vi "Drive Controller.vi"(8 "error in":errorcluster) -> ()   [LabVIEW 2018]
doc: "This VI executes continuously carrying out the current operation and responding to updates or new operation requests. It will often contain the timing or control code that is difficult to place directly in TeleOp. This VI generally opens all sensors and motors and isolates the rest of the robot code from knowing implementation details of how the operations are carried out."
uses:
  <vilib>/Rock Robotics/WPI/Framework/Completion Status.ctl
  Drive Setpoints.ctl
  Drive Operations.ctl
  <vilib>/Rock Robotics/WPI/SafetyOutput/WPI_SafetyOutputConfigMenu.ctl
  <vilib>/Rock Robotics/WPI/RobotDrive/WPI_RobotDriveOpen2MotorWithExistingMotors.vi
  <vilib>/Rock Robotics/Network Tables/NT Write Number.vi
panel:
  in  "Interactive Values":T1
  in  "Buttons":cluster{"Execute Cmd":bool, "Abort Cmd":bool}
  out "Command Timing":cluster{"Start Time (ms)":u32, "Iterations":i32}
  out "Status":T3
  out "Setpoints":T4(graph)
  out "Current\nCmd":string
  # "Tip: The graph shows the motor setpoints. It may also be helpful to observe inputs and sensor values.\nYou may also want to display tuning or debugging controls."
  # "Interactive Command: You may fill in the settings for a command\nand schedule it with the Execute button. You can observe and abort\nany command while fine tuning the code for the controller."
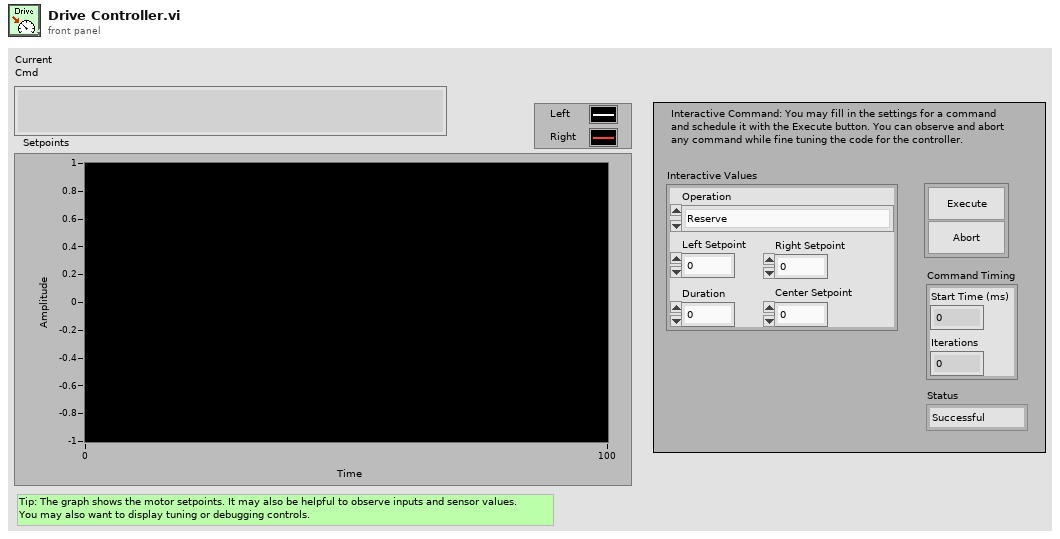
[diagram p1: front panel]
types:
  T1 = typedef "Drive Setpoints.ctl" = cluster{"Operation":T2, "Left Setpoint":dbl, "Right Setpoint":dbl, "Duration":dbl, "Center Setpoint":dbl}
  T2 = typedef "Drive Operations.ctl" = enum16{"Reserve", "Read Current", "Immediate", "Drive for Time", "Drive for Distance"}
  T3 = typedef "Completion Status.ctl" = enum16{"Successful", "Aborted", "Incomplete"}
  T4 = cluster{"Don't move motors while reserved":dbl, "Don't move motors while reserved":dbl, "Center Setpoint":dbl}
  T5 = typedef "WPI_SafetyOutputConfigMenu.ctl" = enum16{"Enable", "Disable"}
  T6 = typedef "WPI_MotorControlDeviceRef.ctl" = cluster{"DeviceStatus":errorcluster, "Type":T7, "PWM":cluster{"PWM Channel":T8, "DeadBand":T9}, "CAN":cluster{"Device Number":u8, "SetOutput VI Ref":variant, "GetOutput VI Ref":variant, "Enable VI Ref":variant, "Disable VI Ref":variant, "Data":variant}, "Invert":bool, "DIO PWM":cluster{"PWM \"Enable\" Channel":T8, "DIOChannel":T10, "PWM Rate":dbl}}
  T7 = typedef "WPI_MotorControlType.ctl" = enum16{"PWM", "CAN", "DIO PWM"}
  T8 = typedef "FPGA_DIOPWMChannel.ctl" = enum8{"PWM 0", "PWM 1", "PWM 2", "PWM 3", "PWM 4", "PWM 5", "PWM 6", "PWM 7", "PWM 8", "PWM 9", "PWM MXP 0", "PWM MXP 1", "PWM MXP 2", "PWM MXP 3", "PWM MXP 4", "PWM MXP 5", "PWM MXP 6", "PWM MXP 7", "PWM MXP 8", "PWM MXP 9", "Invalid"}
  T9 = typedef "WPI_PWMDeadband.ctl" = cluster{"Name":string, "maxPositivePwm":i32, "minPositivePwm":i32, "centerPwm":i32, "maxNegativePwm":i32, "minNegativePwm":i32, "angularRange":u16}
  T10 = typedef "FPGA_DIOChannel.ctl" = enum8{"DIO 0", "DIO 1", "DIO 2", "DIO 3", "DIO 4", "DIO 5", "DIO 6", "DIO 7", "DIO 8", "DIO 9", "DIO MXP 0", "DIO MXP 1", "DIO MXP 2", "DIO MXP 3", "DIO MXP 4", "DIO MXP 5", "DIO MXP 6", "DIO MXP 7", "DIO MXP 8", "DIO MXP 9", "DIO MXP 10", "DIO MXP 11", "DIO MXP 12", "DIO MXP 13", "DIO MXP 14", "DIO MXP 15", "SPI Port CS1", "SPI Port CS2", "SPI Port CS3", "SPI Port MISO", "SPI Port MOSI", "Invalid"}
  T11 = typedef "WPI_RobotDriveDevRef.ctl" = cluster{"DevStatus":errorcluster, "Motors[]":T6[], "Square Inputs":bool, "Max Output":dbl}
  T12 = typedef "Command Status Info.ctl" = cluster{"Name":string, "Status":T3, "notifier out":T13}
  T13 = typedef "Completion Notifier.ctl" = refnum<notifier>
  T14 = cluster{"SubSystem Data":T1, cluster{"Start Time (ms)":u32, "Iterations":i32}, cluster{"Command Info":T12, "Description":string, "Default Command":T1, "queue out":refnum<queue>, "Subsystem Name":string}}
  T15 = cluster{"Yaw":dbl, "Roll":dbl, "Pitch":dbl, "Heading":dbl, "Fused Heading":dbl}
  T16 = cluster{"LinearAcceleration X":dbl, "LinearAcceleration Y":dbl, "LinearAcceleration Z":dbl}
  T17 = cluster{"SubSystem Data":T1, cluster{"Start Time (ms)":u32, "Iterations":i32}, "Default Command Arguments":cluster{"Command Info":T12, "Description":string, "Default Command":T1, "queue out":refnum<queue>, "Subsystem Name":string}}
  T18 = cluster{"Don't move motors while reserved":dbl, "Don't move motors while reserved":dbl, "Don't move motors while reserved":dbl}
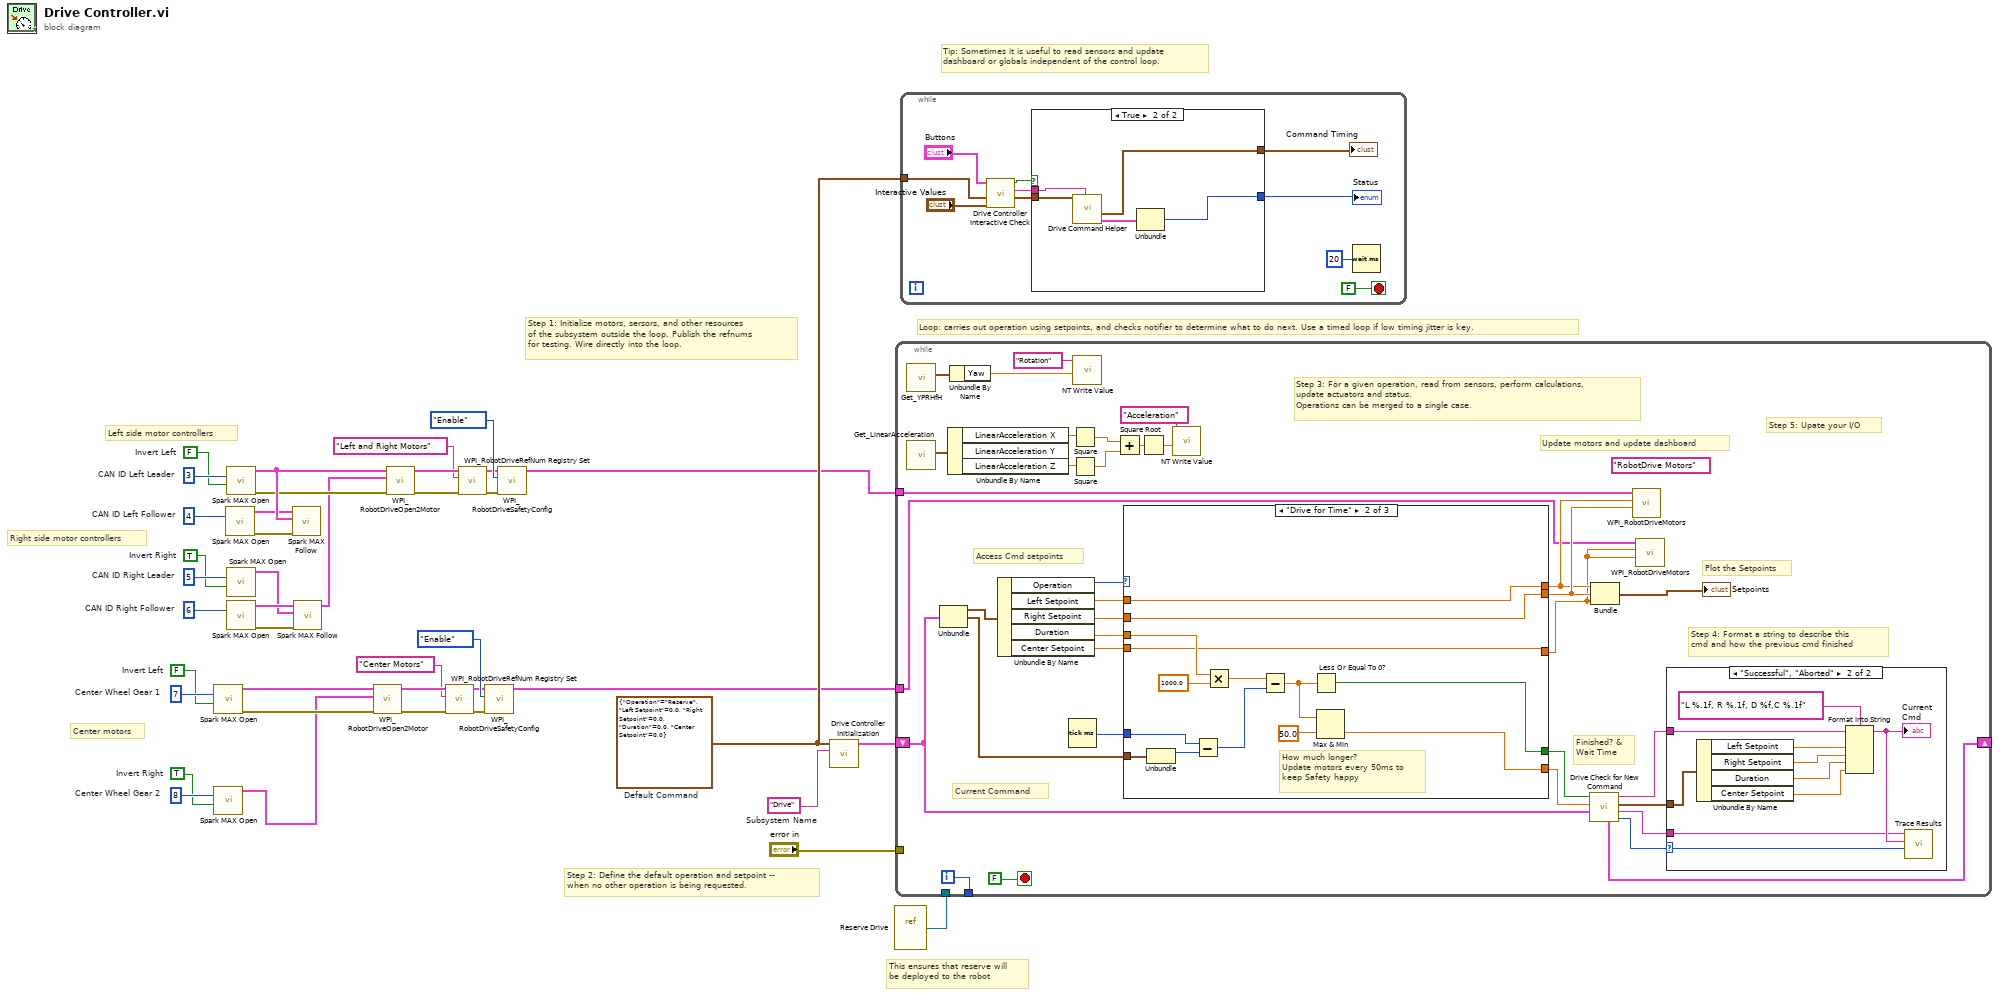
[diagram p0: block diagram]
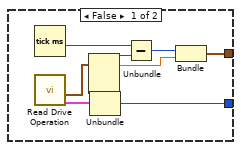
[diagram p2: hidden frame]
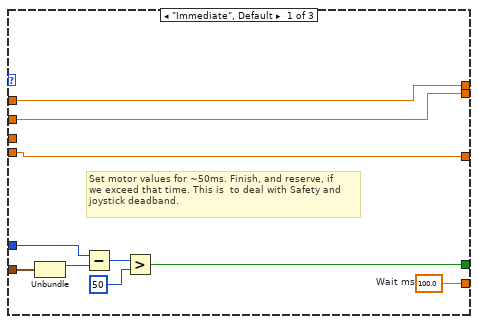
[diagram p4: hidden frame]
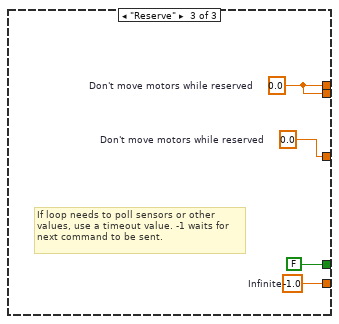
[diagram p5: hidden frame]
diagram:
  w3 = FALSE  # Invert Left
  w4 = TRUE  # Invert Right
  w11 = u8 8  # Center Wheel Gear 2
  w14 = u8 7  # Center Wheel Gear 1
  w16 = FALSE  # Invert Left
  w17 = TRUE  # Invert Right
  w26 = u8 5  # CAN ID Right Leader
  w25 = u8 6  # CAN ID Right Follower
  w34 = u8 3  # CAN ID Left Leader
  w35 = u8 4  # CAN ID Left Follower
  w36 = T1 {"Operation"=enum."Reserve", "Left Setpoint"=0.0, "Right Setpoint"=0.0, "Duration"=0.0, "Center Setpoint"=0.0}  # Default Command
  w40 = "Drive"  # Subsystem Name
  # "Center motors"
  # "Right side motor controllers"
  # "Left side motor controllers"
  # "This ensures that reserve will\nbe deployed to the robot"
  # "Tip: Sometimes it is useful to read sensors and update\ndashboard or globals independent of the control loop."
  # "Step 2: Define the default operation and setpoint --\nwhen no other operation is being requested."
  # "Step 1: Initialize motors, sersors, and other resources\nof the subsystem outside the loop. Publish the refnums\nfor testing. Wire directly into the loop."
  # "Loop: carries out operation using setpoints, and checks notifier to determine what to do next. Use a timed loop if low timing jitter is key."
  n1 = call <vilib>:"Spark MAX Open.vi"("Invert"=w3, "Device Number"=w14) -> ("error out"=w12:errorcluster, "MotorControlDeviceRef"=w13:T6)  [unwired: 8 in]
  n2 = call <vilib>:"Spark MAX Open.vi"("Invert"=w4, "Device Number"=w11) -> ("MotorControlDeviceRef"=w2:T6)  [unwired: 8 in, 1 out]
  n3 = call <vilib>:"Spark MAX Open.vi"("Device Number"=w35) -> ("error out"=w30:errorcluster, "MotorControlDeviceRef"=w31:T6)  [unwired: 9 in]
  n4 = call <vilib>:"Spark MAX Open.vi"("Invert"=w16, "Device Number"=w34) -> ("error out"=w32:errorcluster, "MotorControlDeviceRef"=w33:T6)  [unwired: 8 in]
  n5 = call <vilib>:"Spark MAX Open.vi"("Invert"=w17, "Device Number"=w26) -> ("MotorControlDeviceRef"=w27:T6)  [unwired: 8 in, 1 out]
  n6 = call <vilib>:"Spark MAX Open.vi"("Device Number"=w25) -> ("error out"=w29:errorcluster, "MotorControlDeviceRef"=w28:T6)  [unwired: 9 in]
  n7 = call <vilib>:"Spark MAX Follow.vi"("error in (no error)"=w30, "Master Controller"=w33, "MotorControlDeviceRef"=w31) -> ()  [unwired: 7 in, 2 out]
  n8 = call <vilib>:"Spark MAX Follow.vi"("error in (no error)"=w29, "Master Controller"=w27, "MotorControlDeviceRef"=w28) -> ("MotorControlDeviceRef"=w24:T6)  [unwired: 7 in, 1 out]
  n9 = call-poly <vilib>:"WPI_RobotDriveOpen2Motor.vi"("error in (no error)"=w12, "Right Motor Dev Ref"=w2, "Left Motor Dev Ref"=w13) -> ("error out"=w8:errorcluster, "RobotDriveDevRef"=w10:T11)  [unwired: 7 in]
  n10 = call-poly <vilib>:"WPI_RobotDriveOpen2Motor.vi"("error in (no error)"=w32, "Right Motor Dev Ref"=w24, "Left Motor Dev Ref"=w33) -> ("error out"=w21:errorcluster, "RobotDriveDevRef"=w23:T11)  [unwired: 7 in]
  n11 = call <vilib>:"WPI_RobotDriveRefNum Registry Set.vi"("error in (no error)"=w8, "refnum name"="Center Motors", "RobotDriveDevRef"=w10) -> ("error out"=w5:errorcluster, "RobotDriveDevRef"=w6:T11)  [unwired: 7 in]
  n12 = call <vilib>:"WPI_RobotDriveRefNum Registry Set.vi"("error in (no error)"=w21, "refnum name"="Left and Right Motors", "RobotDriveDevRef"=w23) -> ("error out"=w18:errorcluster, "RobotDriveDevRef"=w19:T11)  [unwired: 7 in]
  n13 = call <vilib>:"WPI_RobotDriveSafetyConfig.vi"("error in (no error)"=w5, "mode"=WPI_SafetyOutputConfigMenu."Enable", "RobotDriveDevRef"=w6) -> ("RobotDriveDevRef"=w1:T11)  [unwired: 7 in, 1 out]
  n14 = call <vilib>:"WPI_RobotDriveSafetyConfig.vi"("error in (no error)"=w18, "mode"=WPI_SafetyOutputConfigMenu."Enable", "RobotDriveDevRef"=w19) -> ("RobotDriveDevRef"=w15:T11)  [unwired: 7 in, 1 out]
  n15 = call "Drive Controller Initialization.vi"("Subsystem Name"=w40, "Default Command"=w36) -> ("Current Command"=w38:T14)  [unwired: 9 in]
  n16 = vi-ref "Reserve Drive.vi"() -> (w37:refnum<vi>)
  n17 = while {
    shift-right: [w63] -> _
    shift-left: w38 -> [w56]
    tunnel: [w74] -> _
    tunnel: w15 -> [w71]
    tunnel: "error in" -> [_]
    tunnel: w37 -> [_]
    tunnel: w1 -> [w53]
    i -> [w74]
    stop <- FALSE stop-if-true
    (unwired) "RobotDrive Motors" ("Name")
    # "Step 5: Upate your I/O"
    # "Step 4: Format a string to describe this\ncmd and how the previous cmd finished"
    # "Current Command"
    # "Update motors and update dashboard"
    # "Plot the Setpoints"
    # "Access Cmd setpoints"
    # "Finished? &\nWait Time"
    # "Step 3: For a given operation, read from sensors, perform calculations,\nupdate actuators and status.\nOperations can be merged to a single case."
    n18 = call <vilib>:"Get_YPRHfH.vi"() -> ("YRPHfH"=w51:T15)  [unwired: 11 in]
    n19 = call <vilib>:"Get_LinearAcceleration.vi"() -> ("Linear Acceleration"=w50:T16)  [unwired: 11 in]
    n20 = Unbundle(w56) -> ("SubSystem Data"=w70:T1, w57:cluster{"Start Time (ms)":u32, "Iterations":i32})  [unwired: 1 out]
    n21 = Unbundle By Name(w50) -> ("LinearAcceleration X"=w44:dbl, "LinearAcceleration Z"=w43:dbl)  [unwired: 1 out]
    n22 = Unbundle By Name(w51) -> ("Yaw"=w47:dbl)
    n23 = Unbundle By Name(w70) -> ("Operation"=w69:T2, "Left Setpoint"=w68:dbl, "Right Setpoint"=w67:dbl, "Duration"=w66:dbl, "Center Setpoint"=w54:dbl)
    n24 = Tick Count (ms)() -> (millisecond timer value=w65:u32)
    n25 = Square(x=w44) -> (x^2=w41:dbl)
    n26 = Square(x=w43) -> (x^2=w42:dbl)
    n27 = call-poly <vilib>:"NT Write Value.vi"("Numeric"=w47, "Name"="Rotation") -> ()  [unwired: 9 in, 1 out]
    n28 = Add(x=w41, y=w42) -> (x+y=w45:dbl)
    n29 = case shown="\"Drive for Time\"" w69 {
      tunnel: [w95 w97 w113] -> w62
      tunnel: [w88 w104 FALSE ("ignore previous (F)")] -> w61
      tunnel: w57 -> [w87 w106 _]
      tunnel: [w94 w103 w111] -> w55
      tunnel: [w93 w102 w111] -> w72
      tunnel: w68 -> [w94 w103 _]
      tunnel: w67 -> [w93 w102 _]
      tunnel: w66 -> [_ w101 _]
      tunnel: w65 -> [w89 w100 _]
      tunnel: [w86 w96 w110] -> w52
      tunnel: w54 -> [w86 w96 _]
      frame "Immediate", Default {
        w95 = 100.0  # Wait ms
        # "Set motor values for ~50ms. Finish, and reserve, if\nwe exceed that time. This is  to deal with Safety and\njoystick deadband."
        n30 = Unbundle(w87) -> ("Start Time (ms)"=w90:u32)  [unwired: 1 out]
        n31 = Subtract(x=w89, y=w90) -> (x-y=w91:u32)
        n32 = Greater?(x=w91, y=u8 50 ("Left Motor")) -> (0:w88:bool)
      }
      frame "Drive for Time" {
        # "How much longer?\nUpdate motors every 50ms to\nkeep Safety happy"
        n33 = Unbundle(w106) -> ("Start Time (ms)"=w105:u32)  [unwired: 1 out]
        n34 = Subtract(x=w100, y=w105) -> (x-y=w109:u32)
        n35 = Multiply(x=w101, y=1000.0) -> (x*y=w108:dbl)
        n36 = Subtract(x=w108, y=w109) -> (x-y=w99:dbl)
        n37 = Less Or Equal To 0?(x=w99) -> (x <= 0?=w104:bool)
        n38 = Max & Min(x=w99, y=50.0) -> (min(x,y)=w97:dbl)  [unwired: 1 out]
      }
      frame "Reserve" {
        w110 = 0.0  # Don't move motors while reserved
        w111 = 0.0  # Don't move motors while reserved
        w113 = -1.0  # Infinite
        # "If loop needs to poll sensors or other\nvalues, use a timeout value. -1 waits for\nnext command to be sent."
      }
    }
    n39 = Square Root(x=w45) -> (sqrt(x)=w46:dbl)
    n40 = call-poly <vilib>:"NT Write Value.vi"("Numeric"=w46, "Name"="Acceleration") -> ()  [unwired: 9 in, 1 out]
    n41 = call "Drive Check for New Command.vi"("input cluster"=w56, "Wait time (ms)"=w62, "Finished?"=w61) -> ("Completion"=w64:T3, "Subsystem Name"=w58:string, "Current Command"=w59:T1, "Initial Trace String"=w60:string, "Next Command"=w63:T17)  [unwired: 4 in]
    n42 = Bundle("Don't move motors while reserved"=w55, "Don't move motors while reserved"=w72, "Don't move motors while reserved"=w52) -> (→"Setpoints":T18)  [unwired: 1 in]
    n43 = call <vilib>:"WPI_RobotDriveMotors.vi"("RightSpeed"=w72, "LeftSpeed"=w55, "RobotDriveDevRef"=w71) -> ()  [unwired: 1 in, 8 out]
    n44 = call <vilib>:"WPI_RobotDriveMotors.vi"("RightSpeed"=w52, "LeftSpeed"=w52, "RobotDriveDevRef"=w53) -> ()  [unwired: 1 in, 8 out]
    n45 = case shown="\"Successful\", \"Aborted\"" w64 {
      selector: w64 -> [_ w85]
      tunnel: w60 -> [_ w81]
      tunnel: w59 -> [_ w82]
      tunnel: w58 -> [_ w78]
      frame "Incomplete", Default {
        # "Continuing current command"
      }
      frame "Successful", "Aborted" {
        # "Report and setup for next command"
        n46 = Unbundle By Name(w82) -> ("Left Setpoint"=w83:dbl, "Right Setpoint"=w84:dbl, "Duration"=w79:dbl, "Center Setpoint"=w77:dbl)
        n47 = Format Into String(format string="L %.1f, R %.1f, D %f,C %.1f", initial string=w81, w83, w84, w79, w77) -> (resulting string=w80:string)  [unwired: 1 in, 1 out]
        "Current\nCmd" <- w80
        n48 = call <vilib>:"Trace Results.vi"("Status of previous command"=w85, "Description"=w80, "Subsystem"=w78) -> ()  [unwired: 9 in]
      }
    }
  }
  n49 = while {
    tunnel: w36 -> [w115]
    stop <- FALSE stop-if-true
    n50 = call "Drive Controller Interactive Check.vi"("Interactive Command In"="Interactive Values", "Default Command"=w115, "Buttons"="Buttons") -> ("Interactive Command Out"=w117:T1, "Trace String"=w118:string, "Schedule"=w119:bool)  [unwired: 6 in]
    n51 = case shown="True" w119 {
      tunnel: [w128 w136] -> w120
      tunnel: [w127 w132] -> w121
      tunnel: w118 -> [_ w134]
      tunnel: w117 -> [_ w133]
      frame False {
        n52 = Tick Count (ms)() -> (millisecond timer value=w131:u32)
        n53 = call "Read Drive Operation.vi"() -> ("Command Info"=w125:T12, "SubSystem Data"=w124:T1)  [unwired: 9 in, 1 out]
        n54 = Unbundle(w124) -> ("Operation"=w129:T2, "Left Setpoint"=w126:dbl)  [unwired: 3 out]
        n55 = Unbundle(w125) -> ("Status"=w128:T3)  [unwired: 2 out]
        n56 = Subtract(x=w131, y=w129) -> (x-y=w130:u32)
        n57 = Bundle(w130, "Left Setpoint"=w126) -> (w127:cluster{u32, "Left Setpoint":dbl})  [unwired: 1 in]
      }
      frame True {
        n58 = call "Drive Command Helper.vi"("Description"=w134, "SubSystem Data"=w133) -> ("Command Info Out"=w135:T12, "Command Timing"=w132:cluster{"Start Time (ms)":u32, "Iterations":i32})  [unwired: 7 in, 1 out]
        n59 = Unbundle(w135) -> ("Status"=w136:T3)  [unwired: 2 out]
      }
    }
    "Status" <- w120
    "Command Timing" <- w121
    n60 = Wait (ms)(milliseconds to wait=u32 20) -> ()  [unwired: 1 out]
  }
